vi "ERD HexToNumeric.vi"(8 "Error In":errorcluster, 10 "Read ERD List":T1[](array[typedef])=[{"ERD Number"=8242, "Data Type"=enum."string"}] {"ERD Number" format="%.0x"}, 11 "GEA2 Reference In":refnum<k24>) -> (0 "Error Out":errorcluster, 2 "Number Out":i32, 3 "GEA2 Reference Out":refnum<k24>)   [LabVIEW 2016]
doc: "This VI reads ERD 2032 and tests that it is within specified bounds."
uses:
  Q:/Common/DLLs/GEA3/GeaCommunication.dll
  Common/DLLs/GEA3/GeaCommunication.dll
  Common/LabVIEW GEA2 Toolkit/LabVIEW_GEA2_Toolkit.lvlibp/type defs/Source_Destination.ctl
  Common/LabVIEW GEA2 Toolkit/LabVIEW_GEA2_Toolkit.lvlibp/type defs/ERD Read Data In.ctl
  Common/LabVIEW GEA2 Toolkit/LabVIEW_GEA2_Toolkit.lvlibp/type defs/Data Type.ctl
  Common/LabVIEW GEA2 Toolkit/LabVIEW_GEA2_Toolkit.lvlibp
panel:
  in  "GEA Inputs":T3={"Source"=228, "Destination"=35} {"Destination" format="%.0x"; "Source" format="%.0x"}
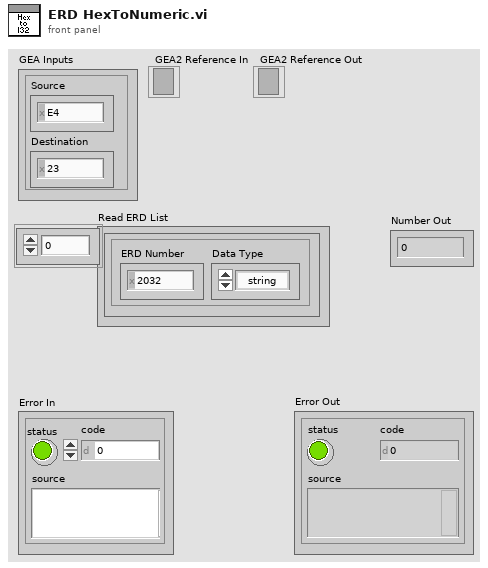
[diagram p1: front panel]
types:
  T1 = typedef "LabVIEW_GEA2_Toolkit.lvlibp/ERD Read Data In.ctl" = cluster{"ERD Number":u16, "Data Type":T2}
  T2 = typedef "LabVIEW_GEA2_Toolkit.lvlibp/Data Type.ctl" = enum16{"string", "boolean", "uint8_t", "uint16_t", "uint32_t", "uint64_t", "int8_t", "int16_t", "int32_t", "int64_t"}
  T3 = typedef "LabVIEW_GEA2_Toolkit.lvlibp/Source_Destination.ctl" = cluster{"Source":u8, "Destination":u8}
  T4 = typedef "LabVIEW_GEA2_Toolkit.lvlibp/ERD Read Data Out.ctl" = cluster{"ERD Number":u16, "Data":string}
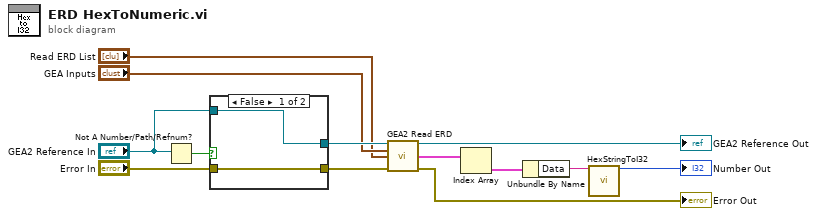
[diagram p0: block diagram]
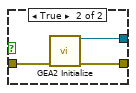
[diagram p2: hidden frame]
diagram:
  n1 = Not A Number/Path/Refnum?(number/path/refnum="GEA2 Reference In") -> (NaN/Path/Refnum?=w11:bool)
  n2 = case shown="False" w11 {
    tunnel: [w15 w18] -> w10
    tunnel: "GEA2 Reference In" -> [w15 _]
    tunnel: "Error In" -> [w14 w17]
    tunnel: [w14 w16] -> w9
    frame False {
    }
    frame True {
      n3 = call "GEA2 Initialize.vi"("error in"=w17) -> ("GEA2 Reference Out"=w18:refnum<k24>, "error out"=w16:errorcluster)  [unwired: 12 in, 1 out]
    }
  }
  n4 = call "GEA2 Read ERD.vi"("GEA2 Reference In"=w10, "GEA Inputs"="GEA Inputs", "Read ERD List"="Read ERD List", "Error In"=w9) -> ("GEA2 Reference Out"=→"GEA2 Reference Out":refnum<k24>, "ERD Data Out"=w6:T4[], "Error Out"=→"Error Out":errorcluster)  [unwired: 8 in, 1 out]
  n5 = Index Array(array=w6) -> (element=w5:T4)  [unwired: 1 in]
  n6 = Unbundle By Name(w5) -> ("Data"=w4:string)
  n7 = call "HexStringToI32.vi"("Input String"=w4) -> ("Number Out"=→"Number Out":i32)  [unwired: 14 in]
